vi "limit_pct.vi"(11 "PCT":dbl) -> (3 "PCT Out":dbl)   [LabVIEW 2011]
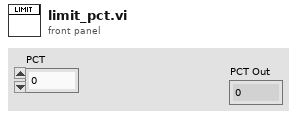
[diagram p1: front panel]
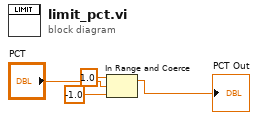
[diagram p0: block diagram]
diagram:
  n1 = In Range and Coerce(upper limit=1.0, x="PCT", lower limit=-1.0) -> (coerced(x)=→"PCT Out":dbl)  [unwired: 1 out]
